vi "WriteStream ClientStreamTemplate.vi"(8 "error in":errorcluster, 10 "Request Data":cluster{"Numeric":dbl}, 11 "Call ID in":T1) -> (0 "error out":errorcluster, 2 "Success":bool, 3 "Call ID":T1)   [LabVIEW 2019, in "Client Template.lvlib"]
uses:
  Client Template.lvlib
  9647bdd3-bda2-4565-bbb9-d670be58a455.vi
  <vilib>/gRPC/LabVIEW gRPC Library/Shared/grpcId.ctl
  <vilib>/gRPC/LabVIEW gRPC Library/grpc-lvsupport-release.lvlib
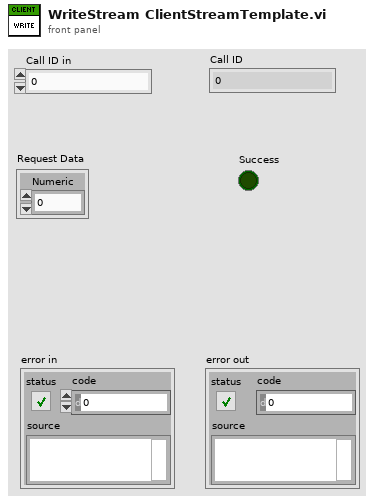
[diagram p1: front panel]
types:
  T1 = typedef "grpc-lvsupport-release.lvlib/grpcId.ctl" = u64
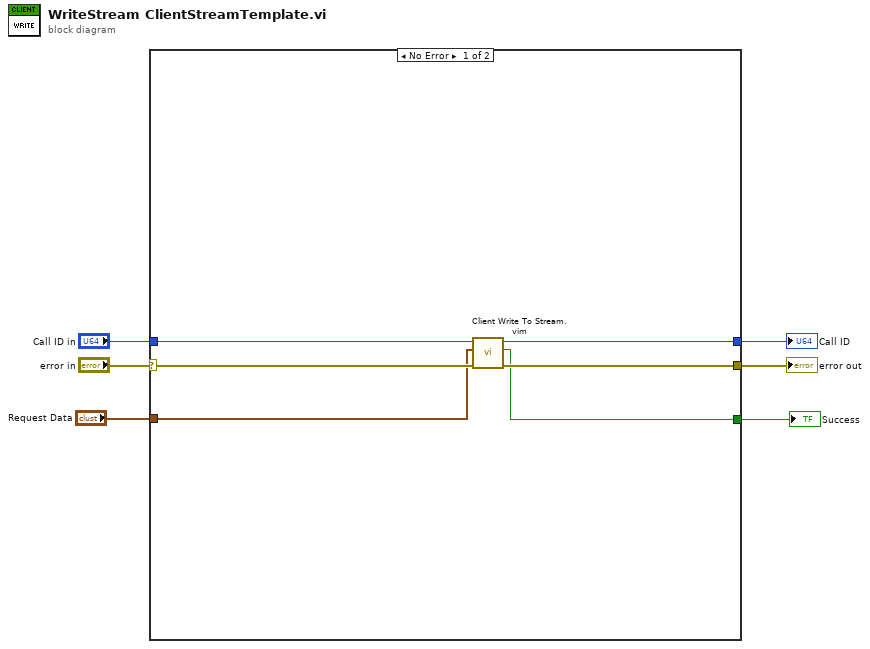
[diagram p0: block diagram]
diagram:
  n1 = case shown="No Error" "error in" {
    selector: "error in" -> [w12 w13]
    tunnel: [w11 w13] -> w5
    tunnel: "Call ID in" -> [w10 w14]
    tunnel: [w9 w14] -> w3
    tunnel: "Request Data" -> [w8 _]
    tunnel: [w7 _] -> w1
    frame No Error {
      n2 = call "Client Write To Stream.vim"("error in"=w12, "Request Data"=w8, "Call ID in"=w10) -> ("error out"=w11:errorcluster, "Success"=w7:bool, "Call ID out"=w9:u64)  [unwired: 6 in]
    }
    frame Error {
    }
  }
  "error out" <- w5
  "Call ID" <- w3
  "Success" <- w1
